vi "Test_Lockin_API.vi"() -> ()   [LabVIEW 2016]
uses:
  RemoteControl/Typedefs/Remote-SMO-Commands-Enum.ctl
  Typedefs/AO-cluster.ctl
  Typedefs/AO_Amp-array.ctl
  Typedefs/AO_DC-array.ctl
  Typedefs/AO_f-array.ctl
  Typedefs/AO_phi-array.ctl
  Typedefs/Function-array.ctl
  Typedefs/Function-enum.ctl
  Typedefs/REF-cluster.ctl
  Typedefs/REF_f-array.ctl
  Typedefs/REF_phi-array.ctl
  <userlib>/_OpenG.lib/error/error.llb/Filter Error Codes (Array)__ogtk.vi
  RemoteControl/LockinRemoteControl.lvclass
panel:
  in  "Tab Control":T1(tab)=enum."config"
  out "getResults":dbl(graph)=-0.0010710766621954784
  in  "disabled index (col)":i32
  in  "disabled index (row)":i32
  out "getAO":waveform(dbl)[](graph)
  out "getAI":waveform(dbl)[](graph)
  in  "Reset":bool
  in  "Keep Taking IV Curves":bool
  in  "Take an IV curve":bool
  in  "Channels: AO":T2={"AO amp (V)"=[0.0, 0.0, 0.0, 0.0, 0.0, 0.0, 0.0, 0.0], "AO DC (V)"=[0.0, 0.0, 0.0, 0.0, 0.0, 0.0, 0.0, 0.0], "AO f (Hz)"=[13.0, 13.0, 13.0, 13.0, 13.0, 13.0, 13.0, 13.0], "AO phi (°)"=[0.0, 0.0, 0.0, 0.0, 0.0, 0.0, 0.0, 0.0], "function"=[enum."Sine", enum."Sine", enum."Sine", enum."Sine", enum."Sine", enum."Sine", enum."Sine", enum."Sine"], "I+"=[]} {"AO f (Hz)" min=0.001 max=10000.0; "AO DC (V)" format="%.3p"; "AO amp (V)" format="%.3p"}
  in  "Channels: Lockin":T9={"REF f (Hz)"=[13.0], "REF phi (°)"=[0.0]} {"REF phi (°)" format="%#_3g"}
  in  "IV mode":bool
  in  "Remote Mode":bool
  in  "Trigger":bool
  out "timeout (ms)":u32=202
  out "IV state counter":u32=1
  in  "side gate channel":i32=1
  in  "phase":dbl
  in  "cycles (1,2,...)":i32=1 min=1 step=1
  in  "Vmin (start)":dbl=-0.15 format="%#_3p"
  in  "Vmax (end)":dbl=0.7 format="%#_3p"
  in  "dV":dbl=0.0005 format="%#_3p"
  in  "function (ramp)":enum16{"Ramp", "Triangle", "Sine"}(ring)
  out "getResults 2":cluster{"Waveform Graph":dbl[], dbl[]}(graph)
  in  "address":string
  in  "Enum":T12
  in  "Stop":bool
  # "1"
  # "2"
  # "3"
  # "4"
  # "5"
  # "6"
  # "7"
  # "8"
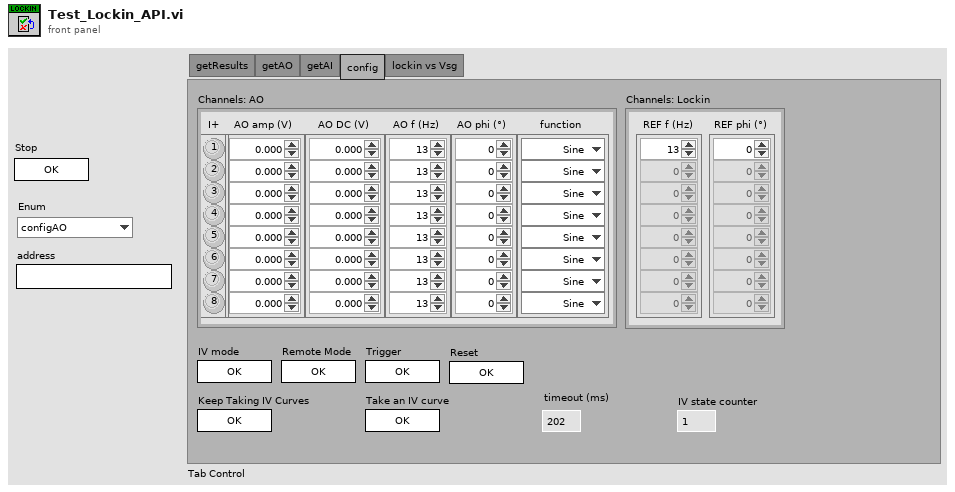
[diagram p1: front panel]
types:
  T1 = enum32{"getResults", "getAO", "getAI", "config", "lockin vs Vsg"}
  T2 = typedef "AO-cluster.ctl" = cluster{"AO amp (V)":T3, "AO DC (V)":T4, "AO f (Hz)":T5, "AO phi (°)":T6, "function":T7, "I+":bool[]}
  T3 = typedef "AO_Amp-array.ctl" = dbl[]
  T4 = typedef "AO_DC-array.ctl" = dbl[]
  T5 = typedef "AO_f-array.ctl" = dbl[]
  T6 = typedef "AO_phi-array.ctl" = dbl[]
  T7 = typedef "Function-array.ctl" = T8[]
  T8 = typedef "Function-enum.ctl" = enum16{"Sine", "Triangle", "Square", "Sawtooth"}
  T9 = typedef "REF-cluster.ctl" = cluster{"REF f (Hz)":T10, "REF phi (°)":T11}
  T10 = typedef "REF_f-array.ctl" = dbl[]
  T11 = typedef "REF_phi-array.ctl" = dbl[]
  T12 = typedef "LockinRemoteControl.lvclass/Remote-SMO-Commands-Enum.ctl" = enum16{"configAO", "configREF", "configREFfilter", "configIVmode", "configRemote", "configReset", "configSampling", "assertTrigger", "getAO", "getAI", "getResults", "getTrigger", "getIVmode", "getSampling", "getAOconfig", "getREFconfig", "getREFfilter", "ACK", "UNK", "CLOSE", "configGain", "getGain"}
  T13 = enum32{"invalid app kind", "Development System", "Run Time System", "Student Edition", "Embedded LabVIEW", "Evaluation", "Custom"}
  T14 = enum32{"Invalid", "Standard", "Closed", "Hidden", "Minimized", "Maximized"}
  T15 = cluster{"Core":cluster{"Current VI Reference":refnum<vi>, "Close Panel on Exit?":bool}, "Your Boolean data":bool, "remote address":string}
  T16 = cluster{"Current VI Reference":refnum<vi>, "Close Panel on Exit?":bool}
  T17 = typedef "LockinRemoteControl.lvclass/PrivateEvents--LockinRemoteControl.setTrigger.ctl" = bool
  T18 = typedef "LockinRemoteControl.lvclass/PrivateEvents--LockinRemoteControl.setIVmode.ctl" = bool
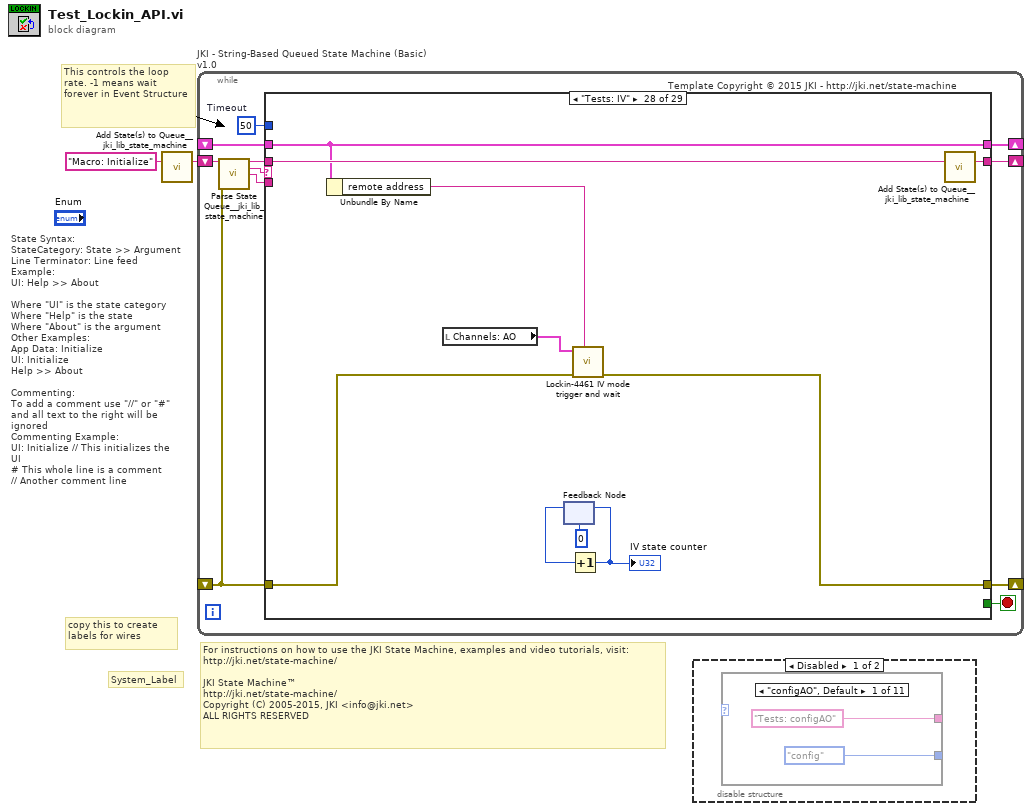
[diagram p0: block diagram]
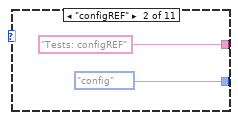
[diagram p2: hidden frame]
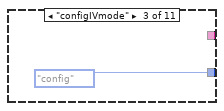
[diagram p3: hidden frame]
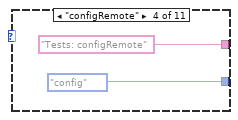
[diagram p4: hidden frame]
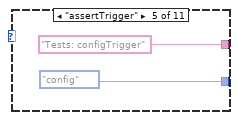
[diagram p5: hidden frame]
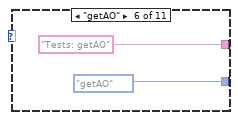
[diagram p6: hidden frame]
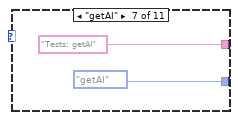
[diagram p7: hidden frame]
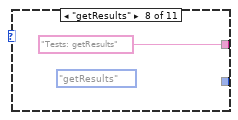
[diagram p8: hidden frame]
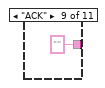
[diagram p9: hidden frame]
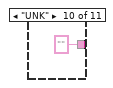
[diagram p10: hidden frame]
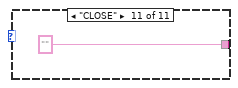
[diagram p11: hidden frame]
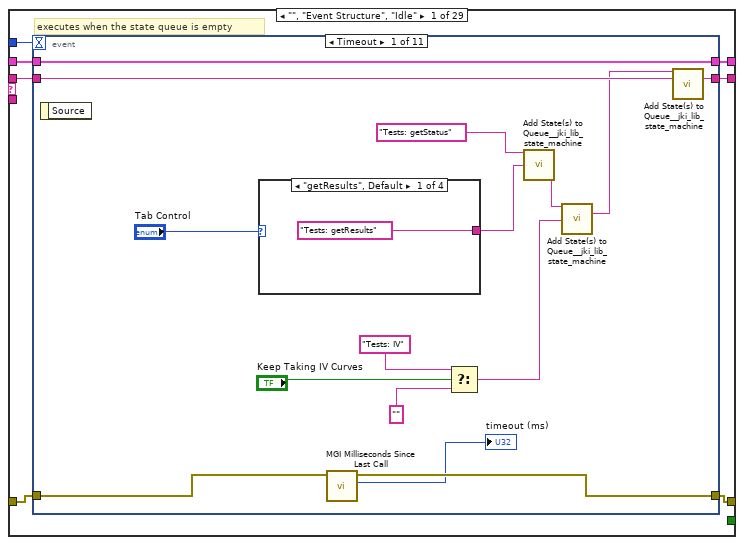
[diagram p13: hidden frame]
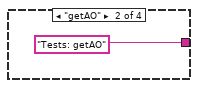
[diagram p14: hidden frame]
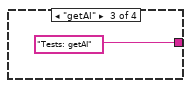
[diagram p15: hidden frame]
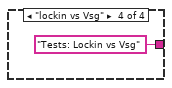
[diagram p16: hidden frame]
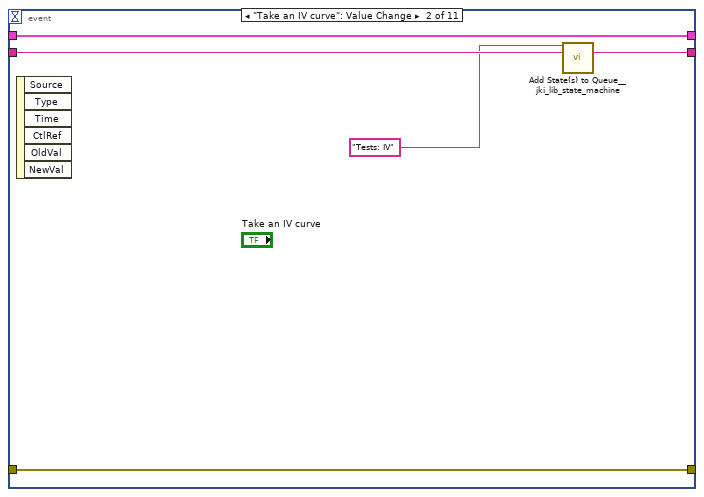
[diagram p17: hidden frame]
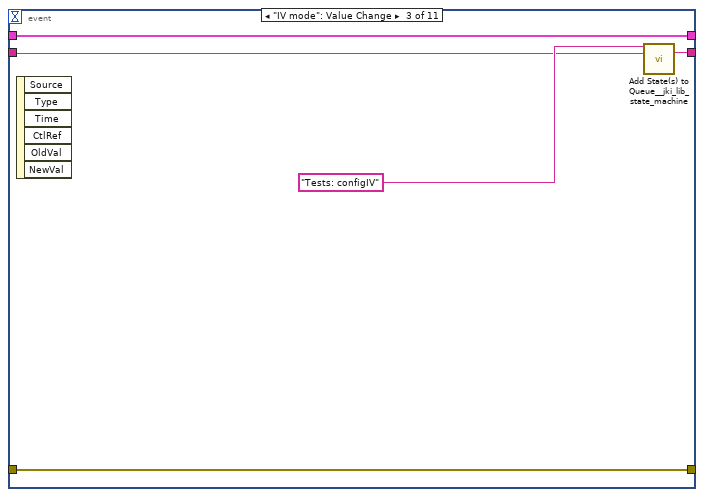
[diagram p18: hidden frame]
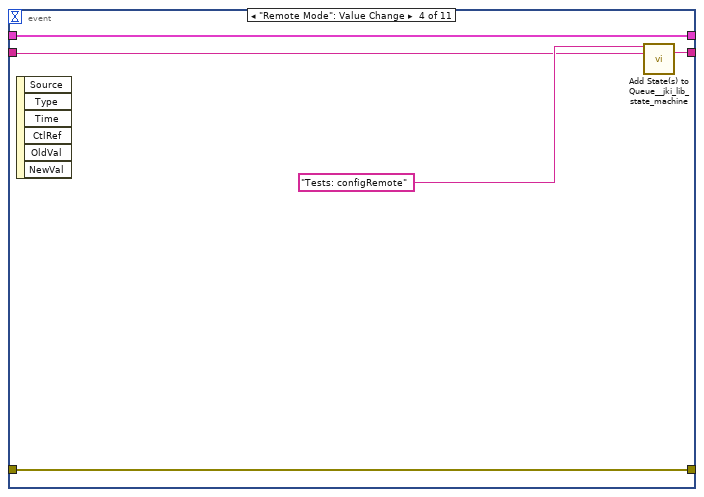
[diagram p19: hidden frame]
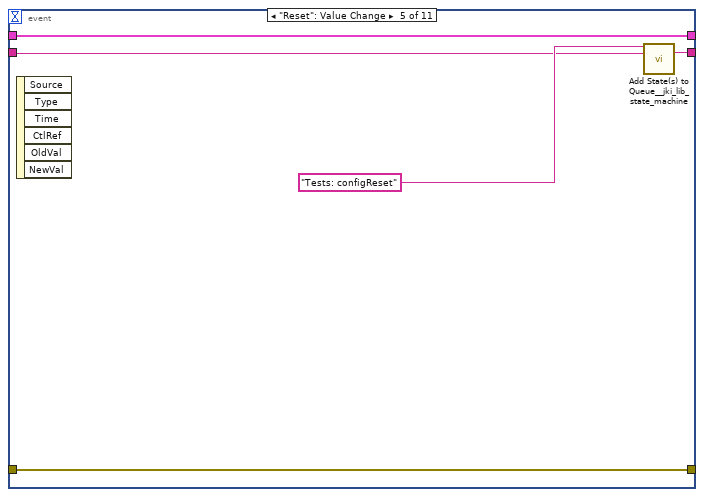
[diagram p20: hidden frame]
diagram:
  # "For instructions on how to use the JKI State Machine, examples and video tutorials, visit:\nhttp://jki.net/state-machine/\n\nJKI State Machine™\nhttp://jki.net/state-machine/\nCopyright (C) 2005-2015, JKI <info@jki.net>\nALL RIGHTS RESERVED"
  # "State Syntax:\nStateCategory: State >> Argument\nLine Terminator: Line feed\nExample:\nUI: Help >> About\n\nWhere \"UI\" is the state category\nWhere \"Help\" is the state\nWhere \"About\" is the argument\nOther Examples:\nApp Data: Initialize\nUI: Initialize\nHelp >> About\n\nCommenting:\nTo add a comment use \"//\" or \"#\" and all text to the right will be ignored\nCommenting Example:\nUI: Initialize // This initializes the UI\n# This whole line is a comment\n// Another comment line"
  # "copy this to create labels for wires"
  # "This controls the loop rate. -1 means wait forever in Event Structure"
  # "System_Label"
  n1 = call <vilib>:"Add State(s) to Queue__jki_lib_state_machine.vi"("State(s) in (\"\")"="Macro: Initialize") -> ("States Out"=w2:string)  [unwired: 14 in]
  n2 = while "JKI - String-Based Queued State Machine (Basic) v1.0" {
    shift-right: [w6] -> _
    shift-left: _ -> [w5]
    shift-right: [w9] -> _
    shift-left: _ -> [w3]
    shift-right: [w8] -> _
    shift-left: w2 -> [w10]
    stop <- w7 stop-if-true
    w4 = 50  # Timeout
    # "Template Copyright © 2015 JKI - http://jki.net/state-machine"
    n3 = call <vilib>:"Parse State Queue__jki_lib_state_machine.vi"("State Queue"=w10, "Error In (no error)"=w3) -> ("Remaining States"=w12:string, "Current State"=w13:string, "Arguments"=w11:string)  [unwired: 11 in]
    n4 = case shown="\"Tests: IV\"" w13 {
      selector: w13 -> [_ _ w94 _ _ _ _ _ _ _ _ _ _ _ _ _ _ _ _ _ _ _ _ _ _ _ _ _ _]
      tunnel: w12 -> [w20 w93 w98 w116 w124 w129 w133 w140 w146 w150 w154 w160 w171 w197 w202 w212 w216 w226 w239 w246 w253 w260 w267 w274 w281 w288 w298 w315 w333]
      tunnel: w11 -> [_ _ _ _ _ _ _ _ _ _ _ w155 w165 _ _ _ _ _ _ _ _ _ _ _ _ _ _ _ _]
      tunnel: w5 -> [w18 w90 w96 w107 w121 w127 w130 _ w141 w147 w152 w158 w167 w194 w199 w209 w213 w219 w237 w241 w248 w255 w262 w269 w276 w286 w294 w310 w321]
      tunnel: [w17 w91 w100 w113 errorcluster {"status"=FALSE, "code"=0, "source"=""} ("error out") w126 w131 w137 w142 w148 w151 w156 w168 w195 w200 w210 w214 w220 w231 w243 w250 w257 w264 w271 w278 w283 w293 w308 w331] -> w9
      tunnel: w3 -> [w16 w91 w99 w113 w119 w126 w131 w137 w143 w148 w151 w157 w169 w195 w200 w210 w214 w221 w234 w244 w251 w258 w265 w272 w279 w284 w296 w309 w331]
      tunnel: [w19 w92 w97 w115 w123 w128 w132 w139 w145 w149 w153 w159 w170 w196 w201 w211 w215 w225 w238 w245 w252 w259 w266 w273 w280 w287 w297 w314 w332] -> w8
      tunnel: [_ _ _ _ _ TRUE _ _ _ _ _ _ _ _ _ _ _ _ _ _ _ _ _ _ _ _ _ _ _] -> w7
      tunnel: [w15 w90 w96 w114 w121 w127 w130 w138 w141 w147 w152 w158 w167 w194 w199 w209 w213 w219 w237 w241 w248 w255 w262 w269 w276 w286 w294 w310 w321] -> w6
      tunnel: w4 -> [w14 _ _ _ _ _ _ _ _ _ _ _ _ _ _ _ _ _ _ _ _ _ _ _ _ _ _ _ _]
      frame "", "Event Structure", "Idle" {
        # "executes when the state queue is empty"
        n5 = event shown="[0] Timeout" {
          selector: _ -> [_ _ _ _ _ _ _ _ _ _ _]
          dyn-events: _ -> [_ _ _ _ _ _ _ _ _ _ _]
          timeout: w14 -> [_ _ _ _ _ _ _ _ _ _ _]
          tunnel: w20 -> [w35 w41 w45 w50 w55 w60 _ _ w77 w83 w89]
          tunnel: [w34 w42 w49 w54 w59 w64 w68 w72 w78 w82 w88] -> w19
          tunnel: w18 -> [w33 w44 w46 w51 w56 w61 w66 w70 w75 w80 w86]
          tunnel: [w22 w43 w47 w52 w57 w62 w67 w71 w76 w81 w87] -> w17
          tunnel: w16 -> [w23 w43 w47 w52 w57 w62 w67 w71 w76 w81 w87]
          tunnel: [w33 w44 w46 w51 w56 w61 w66 w70 w74 w80 w86] -> w15
          event Timeout {
            n6 = event-data() -> ()  [unwired: 1 in, 1 out]
            n7 = case shown="\"getResults\", Default" "Tab Control" {
              tunnel: ["Tests: getResults" "Tests: getAO" "Tests: getAI" "Tests: Lockin vs Vsg"] -> w31
              frame "getResults", Default {
              }
              frame "getAO" {
              }
              frame "getAI" {
              }
              frame "lockin vs Vsg" {
              }
            }
            n8 = call <userlib>:"MGI Milliseconds Since Last Call.vi"("Error In"=w23) -> ("ms"=→"timeout (ms)":u32, "Error Out"=w22:errorcluster)  [unwired: 5 in]
            n9 = Select(t="Tests: IV", s="Keep Taking IV Curves", f="") -> (s? t:f=w24:string)
            n10 = call <vilib>:"Add State(s) to Queue__jki_lib_state_machine.vi"("State(s) in Front (\"\")"="Tests: getStatus", "State(s) at Back (\"\")"=w31) -> ("States Out"=w29:string)  [unwired: 13 in]
            n11 = call <vilib>:"Add State(s) to Queue__jki_lib_state_machine.vi"("State(s) in Front (\"\")"=w29, "State(s) at Back (\"\")"=w24) -> ("States Out"=w28:string)  [unwired: 13 in]
            n12 = call <vilib>:"Add State(s) to Queue__jki_lib_state_machine.vi"("State(s) in Front (\"\")"=w28, "State(s) in (\"\")"=w35) -> ("States Out"=w34:string)  [unwired: 13 in]
          }
          event "Take an IV curve": Value Change {
            n13 = event-data() -> ()  [unwired: 1 in, 6 out]
            n14 = call <vilib>:"Add State(s) to Queue__jki_lib_state_machine.vi"("State(s) in Front (\"\")"="Tests: IV" ("State(s) in Front (\"\")"), "State(s) in (\"\")"=w41) -> ("States Out"=w42:string)  [unwired: 13 in]
          }
          event "IV mode": Value Change {
            n15 = event-data() -> ()  [unwired: 1 in, 6 out]
            n16 = call <vilib>:"Add State(s) to Queue__jki_lib_state_machine.vi"("State(s) in Front (\"\")"="Tests: configIV", "State(s) in (\"\")"=w45) -> ("States Out"=w49:string)  [unwired: 13 in]
          }
          event "Remote Mode": Value Change {
            n17 = event-data() -> ()  [unwired: 1 in, 6 out]
            n18 = call <vilib>:"Add State(s) to Queue__jki_lib_state_machine.vi"("State(s) in Front (\"\")"="Tests: configRemote", "State(s) in (\"\")"=w50) -> ("States Out"=w54:string)  [unwired: 13 in]
          }
          event "Reset": Value Change {
            n19 = event-data() -> ()  [unwired: 1 in, 6 out]
            n20 = call <vilib>:"Add State(s) to Queue__jki_lib_state_machine.vi"("State(s) in Front (\"\")"="Tests: configReset", "State(s) in (\"\")"=w55) -> ("States Out"=w59:string)  [unwired: 13 in]
          }
          event "Trigger": Value Change {
            n21 = event-data() -> ()  [unwired: 1 in, 6 out]
            n22 = call <vilib>:"Add State(s) to Queue__jki_lib_state_machine.vi"("State(s) in Front (\"\")"="Tests: configTrigger", "State(s) in (\"\")"=w60) -> ("States Out"=w64:string)  [unwired: 13 in]
          }
          event Value Change {
            n23 = event-data() -> ()  [unwired: 1 in, 6 out]
            n24 = call <vilib>:"Add State(s) to Queue__jki_lib_state_machine.vi"("State(s) in (\"\")"="Tests: configAO") -> ("States Out"=w68:string)  [unwired: 14 in]
          }
          event Value Change {
            n25 = event-data() -> ()  [unwired: 1 in, 6 out]
            n26 = call <vilib>:"Add State(s) to Queue__jki_lib_state_machine.vi"("State(s) in (\"\")"="Tests: configREF") -> ("States Out"=w72:string)  [unwired: 14 in]
          }
          event "address": Value Change {
            n27 = event-data() -> ()  [unwired: 1 in, 6 out]
            n28 = Bundle By Name(cluster=w75, "remote address"="address") -> (w74:T15)
            n29 = call <vilib>:"Add State(s) to Queue__jki_lib_state_machine.vi"("State(s) in (\"\")"=w77) -> ("States Out"=w78:string)  [unwired: 14 in]
          }
          event "Stop": Value Change {
            # "Exit Button Value Change (pressed) Event\n(this executes Macro: Exit to terminate the VI)"
            n30 = event-data() -> ()  [unwired: 1 in, 1 out]
            n31 = call <vilib>:"Add State(s) to Queue__jki_lib_state_machine.vi"("State(s) in Front (\"\")"="Macro: Exit", "State(s) in (\"\")"=w83) -> ("States Out"=w82:string)  [unwired: 13 in]
          }
          event Panel Close? {
            # "Discard the event because we'll close the front panel ourselves in Macro: Exit"
            # "Close Panel button (pressed) Event\n(this executes Macro: Exit to terminate the VI)"
            n32 = event-data() -> ()  [unwired: 1 in, 1 out]
            n33 = event-data("Discard?"=TRUE) -> ()  [unwired: 1 in, 1 out]
            n34 = call <vilib>:"Add State(s) to Queue__jki_lib_state_machine.vi"("State(s) in Front (\"\")"="Macro: Exit", "State(s) in (\"\")"=w89) -> ("States Out"=w88:string)  [unwired: 13 in]
          }
        }
      }
      frame "---------- Core ----------" {
        # "Do not put any code in this frame.\n(it is a separator no-op)"
        n35 = call <vilib>:"Add State(s) to Queue__jki_lib_state_machine.vi"("State(s) in (\"\")"=w93) -> ("States Out"=w92:string)  [unwired: 14 in]
      }
      frame Default {
        w103 = 42 items=["No error", "Argument error", "Memory is full", "Out of zone", "End of file", "File already open", "Generic file I/O error", "File not found", "File permission error", "Disk is full", "Duplicate path", "Too many files open", "System feature not enabled", "Resource file not found", "Cannot add resource", "Resource not found", "Image not found", "Image memory error", "Pen does not exist", "Config type invalid", "Config token not found", "Config parse error", "Config memory error", "Bad external code format", "Bad external code offset", "External code not present", "Null window", "Destroy window error", "Null menu", "Print aborted", "Bad print record", "Print driver error", "Windows error during printing", "Memory error during printing", "Print dialog error", "Generic print error", "Invalid device refnum", "Device not found", "Device parameter error", "Device unit error", "Cannot open device", "Device call aborted", "Generic error", "Cancelled by user", "Object ID too low", "Object ID too high", "Object not in heap", "Unknown heap", "Unknown object (invalid DefProc)", "Unknown object (DefProc not in table)", "Message out of range", "Invalid (null) method", "Unknown message", "Manager call not supported", "Bad address", "Network operation in progress", "Network operation timed out", "Connection is busy", "Network attribute not supported", "Network error", "Address in use", "System out of memory", "Connection aborted", "Connection refused", "Not connected", "Already connected", "Connection closed", "Initialization error (interapplication manager)", "Bad occurrence", "Wait on unbound occurrence handler", "Occurrence queue overflow", "Datalog type conflict", "Unused", "Unrecognized type (interapplication manager)", "Memory corrupt", "Failed to make temporary DLL", "Old CIN version", "Drag socket not found", "Failed to load drop-object", "Failed to register OLE object", "Failed to release OLE object", "Format specifier type mismatch", "Unknown format specifier", "Too few format specifiers", "Too many format specifiers", "Scan failed", "Newer CIN version", "Error converting to variant", "Runtime menu error", "Password tampered", "Variant attribute not found", "Incompatible variant data type", "Event data is not available", "Event Store is not present", "Occurrence is not found", "Event Queue is not created", "Event info is not available", "Refnum passed is NULL", "Error retrieving Class GUID", "Error retrieving CoClass GUID", "Error retrieving TypeLib GUID.", "Bad built application magic bytes.", "Specific driver is different from the specific driver associated with the Logical Name.", "There is no session opened to the class driver.", "Max Error", "MAX - Error with config objects", "MAX - Error loading configuration", "MAX - Group not supported"]
        # "Current State"
        # "Do not delete, rename, or modify this frame.\n(this is used to capture unhandled states and typos)"
        # "Handle mistyped state name (developer tool)"
        n36 = Format Into String(format string="Software Exception: Unhandled State \"%s\"." ("message"), error in=w99, w94) -> (resulting string=w102:string, error out=w101:errorcluster)  [unwired: 1 in]
        n37 = call <vilib>:"Error Cluster From Error Code.vi"("show call chain? (False)"=TRUE, "error in (no error)"=w101, "error message (\"\")"=w102, "error code (0)"=w103) -> ("error out"=w100:errorcluster)  [unwired: 5 in]
        n38 = call <vilib>:"Add State(s) to Queue__jki_lib_state_machine.vi"("State(s) in (\"\")"=w98) -> ("States Out"=w97:string)  [unwired: 14 in]
      }
      frame "Initialize Core Data" {
        # "Do not delete, rename, or modify this frame.\n(this is used to determine panel behavior on exit)"
        # "originally closed?"
        # "exe?"
        # "If panel starts closed or is an EXE, then close it when we exit"
        n39 = property class="VI"() -> ("Front Panel.Open"=w112:bool)  [unwired: 2 in, 2 out]
        n40 = property class="App"() -> ("App.Kind"=w111:T13)  [unwired: 2 in, 2 out]
        n41 = control-ref of="Current VI Reference"() -> (w105:refnum<vi>)
        n42 = Not(x=w112) -> (.not. x?=w109:bool)
        n43 = Equal?(x=w111, y=T13."Run Time System" ("Application:Kind")) -> (x = y?=w108:bool)
        n44 = Or(x=w109, y=w108) -> (x .or. y?=w106:bool)
        n45 = Bundle By Name(cluster=w107, "Core.Current VI Reference"=w105, "Core.Close Panel on Exit?"=w106) -> (w114:T15)
        n46 = call <vilib>:"Add State(s) to Queue__jki_lib_state_machine.vi"("State(s) in (\"\")"=w116) -> ("States Out"=w115:string)  [unwired: 14 in]
      }
      frame "Error Handler" {
        # "62,63,66 TCP errors\n74 unflatten error resulting from TCP error"
        # "Unhandled Error -- Display it"
        # "Handle any errors here.\nYou can also output any states to clean-up after errors occur"
        # "Clear error"
        n47 = call-poly <userlib>:"Filter Error Codes__ogtk.vi"("Error In"=w119, "Error Codes to Filter"=i32[] [62, 66, 63, 74]) -> ("Error Out"=w118:errorcluster)  [unwired: 7 in, 2 out]
        n48 = call <vilib>:"General Error Handler.vi"("error in (no error)"=w118) -> ()  [unwired: 10 in, 5 out]
        n49 = call <vilib>:"Add State(s) to Queue__jki_lib_state_machine.vi"("State(s) in Front (\"\")"="/* Post Error States", "State(s) in (\"\")"=w124) -> ("States Out"=w123:string)  [unwired: 13 in]
      }
      frame "Exit" {
        # "Do not put any code in this frame.\n(No errors that occur here will be handled.)"
        n50 = call <vilib>:"Add State(s) to Queue__jki_lib_state_machine.vi"("State(s) in (\"\")"=w129) -> ("States Out"=w128:string)  [unwired: 14 in]
      }
      frame "---------- Data ----------" {
        # "Do not put any code in this frame.\n(It is a separator no-op. You can make a copy of this frame to create a new Data frame)"
        n51 = call <vilib>:"Add State(s) to Queue__jki_lib_state_machine.vi"("State(s) in (\"\")"=w133) -> ("States Out"=w132:string)  [unwired: 14 in]
      }
      frame "Data: Initialize" {
        w134 = T16 {"Current VI Reference"=refnum, "Close Panel on Exit?"=FALSE}  # Core
        w136 = TRUE  # Your Boolean data
        w135 = ""  # remote address
        # "do not delete - used by framework"
        # "Expand Bundle to add new data elements to shift register data."
        # "Data names and types of shift register data are defined by this bundle."
        # "Initialize the shift-register data, here.\n(data names are defined by what you wire into the bundle function)"
        n52 = Bundle("Core"=w134, "Your Boolean data"=w136, "remote address"=w135) -> (w138:T15)  [unwired: 1 in]
        n53 = call <vilib>:"Add State(s) to Queue__jki_lib_state_machine.vi"("State(s) in (\"\")"=w140) -> ("States Out"=w139:string)  [unwired: 14 in]
      }
      frame "Data: Cleanup" {
        # "Cleanup any data and references, here.\n(this is called automatically, by the Macro: Exit)"
        n54 = Unbundle By Name(w141) -> ("Core.Current VI Reference"=w144:refnum<vi>)
        n55 = Close Reference(reference=w144, error in (no error)=w143) -> (error out=w142:errorcluster)
        n56 = call <vilib>:"Add State(s) to Queue__jki_lib_state_machine.vi"("State(s) in (\"\")"=w146) -> ("States Out"=w145:string)  [unwired: 14 in]
      }
      frame "---------- UI ----------" {
        # "Do not put any code in this frame.\n(It is a separator no-op. You can make a copy of this frame to create a new UI frame)"
        n57 = call <vilib>:"Add State(s) to Queue__jki_lib_state_machine.vi"("State(s) in (\"\")"=w150) -> ("States Out"=w149:string)  [unwired: 14 in]
      }
      frame "UI: Initialize" {
        # "Initialize the User Interface, here.\n(this is called automatically, by the Macro: Init)"
        n58 = call <vilib>:"Add State(s) to Queue__jki_lib_state_machine.vi"("State(s) in (\"\")"=w154) -> ("States Out"=w153:string)  [unwired: 14 in]
      }
      frame "UI: Cursor Set" {
        # "Argument"
        # "Set and Unset Cursor Busy.\n(Usage: \"UI: Cursor Set >> Busy|Idle\")"
        n59 = case shown="\"Idle\", Default" w155 {
          tunnel: w157 -> [w162 w164]
          tunnel: [w161 w163] -> w156
          frame "Idle", Default {
            n60 = call <vilib>:"Unset Busy.vi"("error in (no error)"=w162) -> ("error out"=w161:errorcluster)  [unwired: 10 in]
          }
          frame "Busy" {
            n61 = call <vilib>:"Set Busy.vi"("error in (no error)"=w164) -> ("error out"=w163:errorcluster)  [unwired: 9 in, 1 out]
          }
        }
        n62 = call <vilib>:"Add State(s) to Queue__jki_lib_state_machine.vi"("State(s) in (\"\")"=w160) -> ("States Out"=w159:string)  [unwired: 14 in]
      }
      frame "UI: Front Panel State" {
        # "Argument"
        # "Set Front Panel Open or Closed\n(Usage: \"UI: Front Panel State >> Open|Close\")"
        n63 = Unbundle By Name(w167) -> ("Core.Current VI Reference"=w166:refnum<vi>)
        n64 = case shown="\"Open\", Default" w165 {
          tunnel: w169 -> [w175 w188]
          tunnel: [w177 w189] -> w168
          tunnel: w166 -> [w176 w186]
          frame "Open", Default {
            n65 = property class="VI"(reference=w176, error in=w175) -> (reference out=w173:refnum<vi>, error out=w174:errorcluster, "Front Panel.Open"=w172:bool)
            n66 = case shown="True" w172 {
              tunnel: [w180 w183] -> w177
              tunnel: w174 -> [w179 w183]
              tunnel: w173 -> [w178 _]
              frame False {
                n67 = invoke class="VI" method="FP.Open"(reference=w178, error in=w179, "Activate"=TRUE, "State"=T14."Standard") -> (error out=w180:errorcluster)  [unwired: 1 in, 4 out]
              }
              frame True {
              }
            }
          }
          frame "Close" {
            n68 = property class="VI"(reference=w186, error in=w188) -> (reference out=w185:refnum<vi>, error out=w187:errorcluster, "Front Panel.Open"=w184:bool)
            n69 = case shown="True" w184 {
              tunnel: [w190 w193] -> w189
              tunnel: w187 -> [w190 w192]
              tunnel: w185 -> [_ w191]
              frame False {
              }
              frame True {
                n70 = invoke class="VI" method="FP.Close"(reference=w191, error in=w192) -> (error out=w193:errorcluster)  [unwired: 1 in, 2 out]
              }
            }
          }
        }
        n71 = call <vilib>:"Add State(s) to Queue__jki_lib_state_machine.vi"("State(s) in (\"\")"=w171) -> ("States Out"=w170:string)  [unwired: 14 in]
      }
      frame "---------- Macro ----------" {
        # "Do not put any code in this frame.\n(It is a separator no-op. You can make a copy of this frame to create a new Macro frame)"
        n72 = call <vilib>:"Add State(s) to Queue__jki_lib_state_machine.vi"("State(s) in (\"\")"=w197) -> ("States Out"=w196:string)  [unwired: 14 in]
      }
      frame "Macro: Initialize" {
        w198 = "Data: Initialize\nInitialize Core Data\nUI: Initialize\nUI: Front Panel State >> Open"  # Data: Initialize Initialize Core Data UI: Initialize UI: Front Panel State >> Open
        # "Initialization Macro\n(This is called once, when the VI starts)"
        n73 = call <vilib>:"Add State(s) to Queue__jki_lib_state_machine.vi"("State(s) in Front (\"\")"=w198, "State(s) in (\"\")"=w202) -> ("States Out"=w201:string)  [unwired: 13 in]
      }
      frame "Macro: Exit" {
        # "Exit Macro\n(This is called once, when the VI exits)"
        n74 = Unbundle By Name(w209) -> ("Core.Close Panel on Exit?"=w208:bool)
        n75 = Select(t="UI: Front Panel State >> Close", s=w208, f="") -> (s? t:f=w205:string)
        n76 = call <vilib>:"Add State(s) to Queue__jki_lib_state_machine.vi"("State(s) in (\"\")"=w205, "State(s) at Back (\"\")"="Data: Cleanup\nExit") -> ("States Out"=w203:string)  [unwired: 13 in]
        n77 = call <vilib>:"Add State(s) to Queue__jki_lib_state_machine.vi"("State(s) in Front (\"\")"=w203, "State(s) in (\"\")"=w212) -> ("States Out"=w211:string)  [unwired: 13 in]
      }
      frame "---------- Tests ----------" {
        # "Template Separator\n(You can make a copy of, or modify, this frame)"
        n78 = call <vilib>:"Add State(s) to Queue__jki_lib_state_machine.vi"("State(s) in (\"\")"=w216) -> ("States Out"=w215:string)  [unwired: 14 in]
      }
      frame "Tests: getResults" {
        n79 = Unbundle By Name(w219) -> ("remote address"=w218:string)
        n80 = call "readResults.vi"("address"=w218, "error in (no error)"=w221) -> ("error out"=w220:errorcluster, "Results"=w217:dbl[][])  [unwired: 7 in, 1 out]
        n81 = Index Array(array=w217, index (row)="disabled index (row)", index (col)="disabled index (col)") -> (element=→"getResults":dbl)
        n82 = call <vilib>:"Add State(s) to Queue__jki_lib_state_machine.vi"("State(s) in (\"\")"=w226) -> ("States Out"=w225:string)  [unwired: 14 in]
      }
      frame "Tests: getStatus" {
        # "Template Separator\n(You can make a copy of, or modify, this frame)"
        n83 = Unbundle By Name(w237) -> ("remote address"=w232:string)
        n84 = call "readTrigger.vi"("address"=w232, "error in (no error)"=w234) -> ("error out"=w236:errorcluster, "Trigger"=w230:T17)  [unwired: 8 in]
        n85 = local write "Trigger"(w230) -> ()
        n86 = call "readAOconfig.vi"("address"=w232, "error in (no error)"=w236) -> ("error out"=w235:errorcluster, "AOconfig"=w229:T2)  [unwired: 8 in]
        n87 = local write "Channels: AO"(w229) -> ()
        n88 = call "readREFconfig.vi"("address"=w232, "error in (no error)"=w235) -> ("error out"=w233:errorcluster, "REFconfig"=w228:T9)  [unwired: 8 in]
        n89 = local write "Channels: Lockin"(w228) -> ()
        n90 = call "readIVmode.vi"("address"=w232, "error in (no error)"=w233) -> ("error out"=w231:errorcluster, "IV mode"=w227:T18)  [unwired: 8 in]
        n91 = local write "IV mode"(w227) -> ()
        n92 = call <vilib>:"Add State(s) to Queue__jki_lib_state_machine.vi"("State(s) in (\"\")"=w239) -> ("States Out"=w238:string)  [unwired: 14 in]
      }
      frame "Tests: getAI" {
        n93 = Unbundle By Name(w241) -> ("remote address"=w242:string)
        n94 = call "readAI.vi"("address"=w242, "error in (no error)"=w244) -> ("error out"=w243:errorcluster, "input signal"=→"getAI":waveform(dbl)[])  [unwired: 8 in]
        n95 = call <vilib>:"Add State(s) to Queue__jki_lib_state_machine.vi"("State(s) in (\"\")"=w246) -> ("States Out"=w245:string)  [unwired: 14 in]
      }
      frame "Tests: getAO" {
        n96 = Unbundle By Name(w248) -> ("remote address"=w249:string)
        n97 = call "readAO.vi"("address"=w249, "error in (no error)"=w251) -> ("error out"=w250:errorcluster, "output signal"=→"getAO":waveform(dbl)[])  [unwired: 8 in]
        n98 = call <vilib>:"Add State(s) to Queue__jki_lib_state_machine.vi"("State(s) in (\"\")"=w253) -> ("States Out"=w252:string)  [unwired: 14 in]
      }
      frame "Tests: configAO" {
        n99 = Unbundle By Name(w255) -> ("remote address"=w256:string)
        n100 = call "configAO.vi"("address"=w256, "error in (no error)"=w258, "Channels: AO in"="Channels: AO") -> ("error out"=w257:errorcluster)  [unwired: 7 in, 1 out]
        n101 = call <vilib>:"Add State(s) to Queue__jki_lib_state_machine.vi"("State(s) in (\"\")"=w260) -> ("States Out"=w259:string)  [unwired: 14 in]
      }
      frame "Tests: configREF" {
        n102 = Unbundle By Name(w262) -> ("remote address"=w263:string)
        n103 = call "configREF.vi"("address"=w263, "error in (no error)"=w265, "Channels: Lockin in"="Channels: Lockin") -> ("error out"=w264:errorcluster)  [unwired: 7 in, 1 out]
        n104 = call <vilib>:"Add State(s) to Queue__jki_lib_state_machine.vi"("State(s) in (\"\")"=w267) -> ("States Out"=w266:string)  [unwired: 14 in]
      }
      frame "Tests: configIV" {
        n105 = Unbundle By Name(w269) -> ("remote address"=w270:string)
        n106 = call "configIVmode.vi"("address"=w270, "error in (no error)"=w272, "IV mode"="IV mode") -> ("error out"=w271:errorcluster)  [unwired: 8 in]
        n107 = call <vilib>:"Add State(s) to Queue__jki_lib_state_machine.vi"("State(s) in (\"\")"=w274) -> ("States Out"=w273:string)  [unwired: 14 in]
      }
      frame "Tests: configRemote" {
        n108 = Unbundle By Name(w276) -> ("remote address"=w277:string)
        n109 = call "configRemote.vi"("address"=w277, "error in (no error)"=w279, "Remote Mode"="Remote Mode") -> ("error out"=w278:errorcluster)  [unwired: 8 in]
        n110 = call <vilib>:"Add State(s) to Queue__jki_lib_state_machine.vi"("State(s) in (\"\")"=w281) -> ("States Out"=w280:string)  [unwired: 14 in]
      }
      frame "Tests: configReset" {
        n111 = Unbundle By Name(w286) -> ("remote address"=w285:string)
        n112 = call "configReset.vi"("address"=w285, "error in (no error)"=w284, "Reset"="Reset") -> ("error out"=w283:errorcluster)  [unwired: 8 in]
        n113 = call <vilib>:"Add State(s) to Queue__jki_lib_state_machine.vi"("State(s) in (\"\")"=w288) -> ("States Out"=w287:string)  [unwired: 14 in]
      }
      frame "Tests: configTrigger" {
        n114 = Unbundle By Name(w294) -> ("remote address"=w295:string)
        n115 = call "assertTrigger.vi"("address"=w295, "error in (no error)"=w296, "Trigger"="Trigger") -> ("error out"=w291:errorcluster)  [unwired: 8 in]
        n116 = call <userlib>:"Tick Count (ms)__ogtk.vi"("error in (no error)"=w291) -> ("error out"=w292:errorcluster, "millisecond timer value"=w290:u32)  [unwired: 9 in]
        n117 = while {
          tunnel: w295 -> [w305]
          shift-right: [w304] -> w293
          shift-left: w292 -> [w302]
          tunnel: w290 -> [w300]
          stop <- w299 continue-if-true
          n118 = call <userlib>:"Tick Count (ms)__ogtk.vi"("error in (no error)"=w302) -> ("error out"=w303:errorcluster, "millisecond timer value"=w301:u32)  [unwired: 9 in]
          n119 = Subtract(x=w301, y=w300) -> ()  [unwired: 1 out]
          n120 = call "readTrigger.vi"("address"=w305, "error in (no error)"=w303) -> ("error out"=w304:errorcluster, "Trigger"=w299:T17)  [unwired: 8 in]
          n121 = local write "Trigger"(w299) -> ()
        }
        n122 = call <vilib>:"Add State(s) to Queue__jki_lib_state_machine.vi"("State(s) in (\"\")"=w298) -> ("States Out"=w297:string)  [unwired: 14 in]
      }
      frame "Tests: IV" {
        n123 = Unbundle By Name(w310) -> ("remote address"=w307:string)
        n124 = local read "Channels: AO"() -> (w306:T2)
        n125 = feedback #1(u32 0) -> (w311:u32)
        n126 = Increment(x=w311) -> (x+1=w313:u32)
        "IV state counter" <- w313
        n127 = feedback-in #1(w313) -> ()
        n128 = call "Lockin-4461 IV mode trigger and wait.vi"("address"=w307, "error in (no error)"=w309, "Channels: AO"=w306) -> ("error out"=w308:errorcluster)  [unwired: 7 in, 1 out]
        n129 = call <vilib>:"Add State(s) to Queue__jki_lib_state_machine.vi"("State(s) in (\"\")"=w315) -> ("States Out"=w314:string)  [unwired: 14 in]
      }
      frame "Tests: Lockin vs Vsg" {
        n130 = Unbundle By Name(w321) -> ("remote address"=w320:string)
        n131 = call <userlib>:"Max_Min_conversion.vi"("Min"="Vmin (start)", "Max"="Vmax (end)") -> ("offset"=w324:dbl, "Amplitude"=w323:dbl)  [unwired: 8 in]
        n132 = local read "Channels: AO"() -> (w316:T2)
        n133 = call <userlib>:"Ramp.vi"("phase"="phase", "function (ramp)"="function (ramp)", "cycles (1,2,...)"="cycles (1,2,...)", "step size"="dV", "offset"=w324, "amplitude"=w323) -> ("Waveform Graph"=w319:dbl[])  [unwired: 3 in, 2 out]
        n134 = for {
          tunnel: w319 -> [w342] mode=indexing
          tunnel: "side gate channel" -> [w341]
          tunnel: w316 -> [w340]
          tunnel: w320 -> [w335]
          tunnel: [w338] -> w318 mode=indexing
          w339 = 0 ("index (row)")
          n135 = call "configAO_DC.vi"("address"=w335, "new DC (V)"=w342, "AO Channel"=w341, "Channels: AO"=w340) -> ("error out"=w337:errorcluster)  [unwired: 6 in, 1 out]
          n136 = call "waitForNewWaveforms.vi"("address"=w335, "error in (no error)"=w337) -> ("error out"=w336:errorcluster)  [unwired: 8 in, 1 out]
          n137 = call "readResults.vi"("address"=w335, "error in (no error)"=w336) -> ("Results"=w334:dbl[][])  [unwired: 7 in, 2 out]
          n138 = Index Array(array=w334, index (row)=w339, index (col)=w339) -> (element=w338:dbl)
        }
        n139 = Bundle("Waveform Graph"=w319, w318) -> (→"getResults 2":cluster{"Waveform Graph":dbl[], dbl[]})  [unwired: 1 in]
        n140 = call <vilib>:"Add State(s) to Queue__jki_lib_state_machine.vi"("State(s) in (\"\")"=w333) -> ("States Out"=w332:string)  [unwired: 14 in]
      }
    }
  }
  n141 = disable-structure shown="Disabled" {
    frame Disabled {
      n142 = case shown="\"configAO\", Default" {
        selector: _ -> [_ _ _ _ _ _ _ _ _ _ _]
        tunnel: ["Tests: configAO" "Tests: configREF" w348 "Tests: configRemote" "Tests: configTrigger" "Tests: getAO" "Tests: getAI" "Tests: getResults" "" "" ""] -> _
        tunnel: [enum32{"getResults", "getAO", "getAI", "config"}."config" ("Tab Control") enum32{"getResults", "getAO", "getAI", "config"}."config" ("Tab Control") enum32{"getResults", "getAO", "getAI", "config"}."config" ("Tab Control") enum32{"getResults", "getAO", "getAI", "config"}."config" ("Tab Control") enum32{"getResults", "getAO", "getAI", "config"}."config" ("Tab Control") enum32{"getResults", "getAO", "getAI", "config"}."getAO" ("Tab Control") enum32{"getResults", "getAO", "getAI", "config"}."getAI" ("Tab Control") _ _ _ _] -> _
        frame "configAO", Default {
        }
        frame "configREF" {
        }
        frame "configIVmode" {
        }
        frame "configRemote" {
        }
        frame "assertTrigger" {
        }
        frame "getAO" {
        }
        frame "getAI" {
        }
        frame "getResults" {
          (unwired) enum32{"getResults", "getAO", "getAI", "config"}."getResults" ("Tab Control")
        }
        frame "ACK" {
        }
        frame "UNK" {
        }
        frame "CLOSE" {
        }
      }
    }
    frame Enabled {
    }
  }
